vi "test-swerve-drve-odometry-02.vi"() -> (3 "Test Passed":bool)   [LabVIEW 2019]
uses:
  <vilib>/Rock Robotics/WPI/ThirdParty/JAS_Junk/TrajLib/SWERVE_DRIVE_ODOMETRY.ctl
  <vilib>/Rock Robotics/WPI/ThirdParty/JAS_Junk/TrajLib/POSE2D.ctl
  <vilib>/Rock Robotics/WPI/ThirdParty/JAS_Junk/TrajLib/TRANSLATION2D.ctl
  <vilib>/Rock Robotics/WPI/ThirdParty/JAS_Junk/TrajLib/ROTATION2D.ctl
  <vilib>/Rock Robotics/WPI/ThirdParty/JAS_Junk/TrajLib/SWERVE_DRIVE_KINEMATICS.ctl
  <vilib>/Analysis/Matrix/Datatypes/RealMatrix.ctl
  <vilib>/Rock Robotics/WPI/ThirdParty/JAS_Junk/TrajLib/Conv_Deg_Radians.vi
  <vilib>/Rock Robotics/WPI/ThirdParty/JAS_Junk/TrajLib/Rotation_CreateAngle.vi
  <vilib>/Rock Robotics/WPI/ThirdParty/JAS_Junk/TrajLib/Trajectory_Library.lvlib
  <vilib>/Analysis/Matrix/NI_Matrix.lvlib
panel:
  out "SWERVE_DRIVE_KINEMATICS":T1 {"PrevCoR"."Y" format="%14.3f"; "PrevCoR"."X" format="%14.3f"; "Modules"."Y" format="%14.3f"; "Modules"."X" format="%14.3f"}
  out "Odom 1":T4={"POSE"={"TRANSLATION"={"X"=0.0, "Y"=0.0}, "ROTATION"={"VALUE"=0.0, "COS"=1.0, "SIN"=0.0}}, "GyroOffset"={"VALUE"=0.0, "COS"=1.0, "SIN"=0.0}, "PreviousAngle"={"VALUE"=0.0, "COS"=1.0, "SIN"=0.0}, "PrevTime"=0.0} {"PreviousAngle"."SIN" format="%13.4f"; "PreviousAngle"."COS" format="%13.4f"; "PreviousAngle"."VALUE" format="%13.4f"; "GyroOffset"."SIN" format="%13.4f"; "GyroOffset"."COS" format="%13.4f"; "GyroOffset"."VALUE" format="%13.4f"; "POSE"."ROTATION"."SIN" format="%13.4f"; "POSE"."ROTATION"."COS" format="%13.4f"; "POSE"."ROTATION"."VALUE" format="%13.4f"; "POSE"."TRANSLATION"."Y" format="%14.3f"; "POSE"."TRANSLATION"."X" format="%14.3f"}
  out "Odom 0":T4={"POSE"={"TRANSLATION"={"X"=0.0, "Y"=0.0}, "ROTATION"={"VALUE"=0.0, "COS"=1.0, "SIN"=0.0}}, "GyroOffset"={"VALUE"=0.0, "COS"=1.0, "SIN"=0.0}, "PreviousAngle"={"VALUE"=0.0, "COS"=1.0, "SIN"=0.0}, "PrevTime"=0.0} {"PreviousAngle"."SIN" format="%13.4f"; "PreviousAngle"."COS" format="%13.4f"; "PreviousAngle"."VALUE" format="%13.4f"; "GyroOffset"."SIN" format="%13.4f"; "GyroOffset"."COS" format="%13.4f"; "GyroOffset"."VALUE" format="%13.4f"; "POSE"."ROTATION"."SIN" format="%13.4f"; "POSE"."ROTATION"."COS" format="%13.4f"; "POSE"."ROTATION"."VALUE" format="%13.4f"; "POSE"."TRANSLATION"."Y" format="%14.3f"; "POSE"."TRANSLATION"."X" format="%14.3f"}
  out "robot POSE 0":T5={"TRANSLATION"={"X"=0.0, "Y"=0.0}, "ROTATION"={"VALUE"=0.0, "COS"=1.0, "SIN"=0.0}} {"ROTATION"."SIN" format="%13.4f"; "ROTATION"."COS" format="%13.4f"; "ROTATION"."VALUE" format="%13.4f"; "TRANSLATION"."Y" format="%14.3f"; "TRANSLATION"."X" format="%14.3f"}
  out "robot POSE 1":T5={"TRANSLATION"={"X"=0.0, "Y"=0.0}, "ROTATION"={"VALUE"=0.0, "COS"=1.0, "SIN"=0.0}} {"ROTATION"."SIN" format="%13.4f"; "ROTATION"."COS" format="%13.4f"; "ROTATION"."VALUE" format="%13.4f"; "TRANSLATION"."Y" format="%14.3f"; "TRANSLATION"."X" format="%14.3f"}
  out "robot POSE 2":T5={"TRANSLATION"={"X"=0.0, "Y"=0.0}, "ROTATION"={"VALUE"=0.0, "COS"=1.0, "SIN"=0.0}} {"ROTATION"."SIN" format="%13.4f"; "ROTATION"."COS" format="%13.4f"; "ROTATION"."VALUE" format="%13.4f"; "TRANSLATION"."Y" format="%14.3f"; "TRANSLATION"."X" format="%14.3f"}
  out "Odom 2":T4={"POSE"={"TRANSLATION"={"X"=0.0, "Y"=0.0}, "ROTATION"={"VALUE"=0.0, "COS"=1.0, "SIN"=0.0}}, "GyroOffset"={"VALUE"=0.0, "COS"=1.0, "SIN"=0.0}, "PreviousAngle"={"VALUE"=0.0, "COS"=1.0, "SIN"=0.0}, "PrevTime"=0.0} {"PreviousAngle"."SIN" format="%13.4f"; "PreviousAngle"."COS" format="%13.4f"; "PreviousAngle"."VALUE" format="%13.4f"; "GyroOffset"."SIN" format="%13.4f"; "GyroOffset"."COS" format="%13.4f"; "GyroOffset"."VALUE" format="%13.4f"; "POSE"."ROTATION"."SIN" format="%13.4f"; "POSE"."ROTATION"."COS" format="%13.4f"; "POSE"."ROTATION"."VALUE" format="%13.4f"; "POSE"."TRANSLATION"."Y" format="%14.3f"; "POSE"."TRANSLATION"."X" format="%14.3f"}
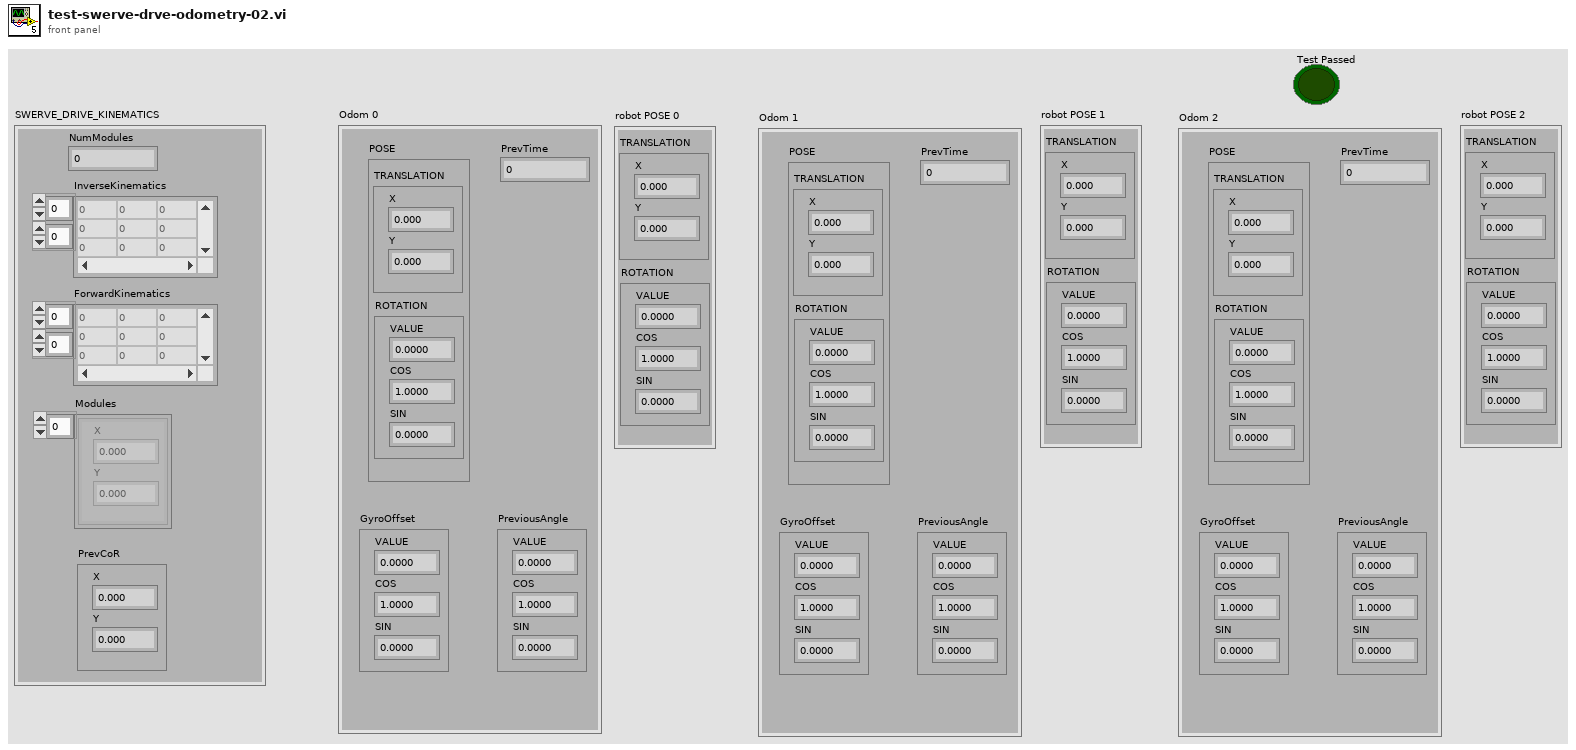
[diagram p1: front panel]
types:
  T1 = typedef "Trajectory_Library.lvlib/SWERVE_DRIVE_KINEMATICS.ctl" = cluster{"NumModules":i32, "InverseKinematics":T2, "ForwardKinematics":T2, "Modules":T3[], "PrevCoR":T3}
  T2 = typedef "NI_Matrix.lvlib/RealMatrix.ctl" = dbl[][]
  T3 = typedef "Trajectory_Library.lvlib/TRANSLATION2D.ctl" = cluster{"X":dbl, "Y":dbl}
  T4 = typedef "Trajectory_Library.lvlib/SWERVE_DRIVE_ODOMETRY.ctl" = cluster{"POSE":T5, "GyroOffset":T6, "PreviousAngle":T6, "PrevTime":dbl}
  T5 = typedef "Trajectory_Library.lvlib/POSE2D.ctl" = cluster{"TRANSLATION":T3, "ROTATION":T6}
  T6 = typedef "Trajectory_Library.lvlib/ROTATION2D.ctl" = cluster{"VALUE":dbl, "COS":dbl, "SIN":dbl}
  T7 = typedef "Trajectory_Library.lvlib/SWERVE_DRIVE_MODULE_STATE.ctl" = cluster{"Speed":dbl, "Angle":T6}
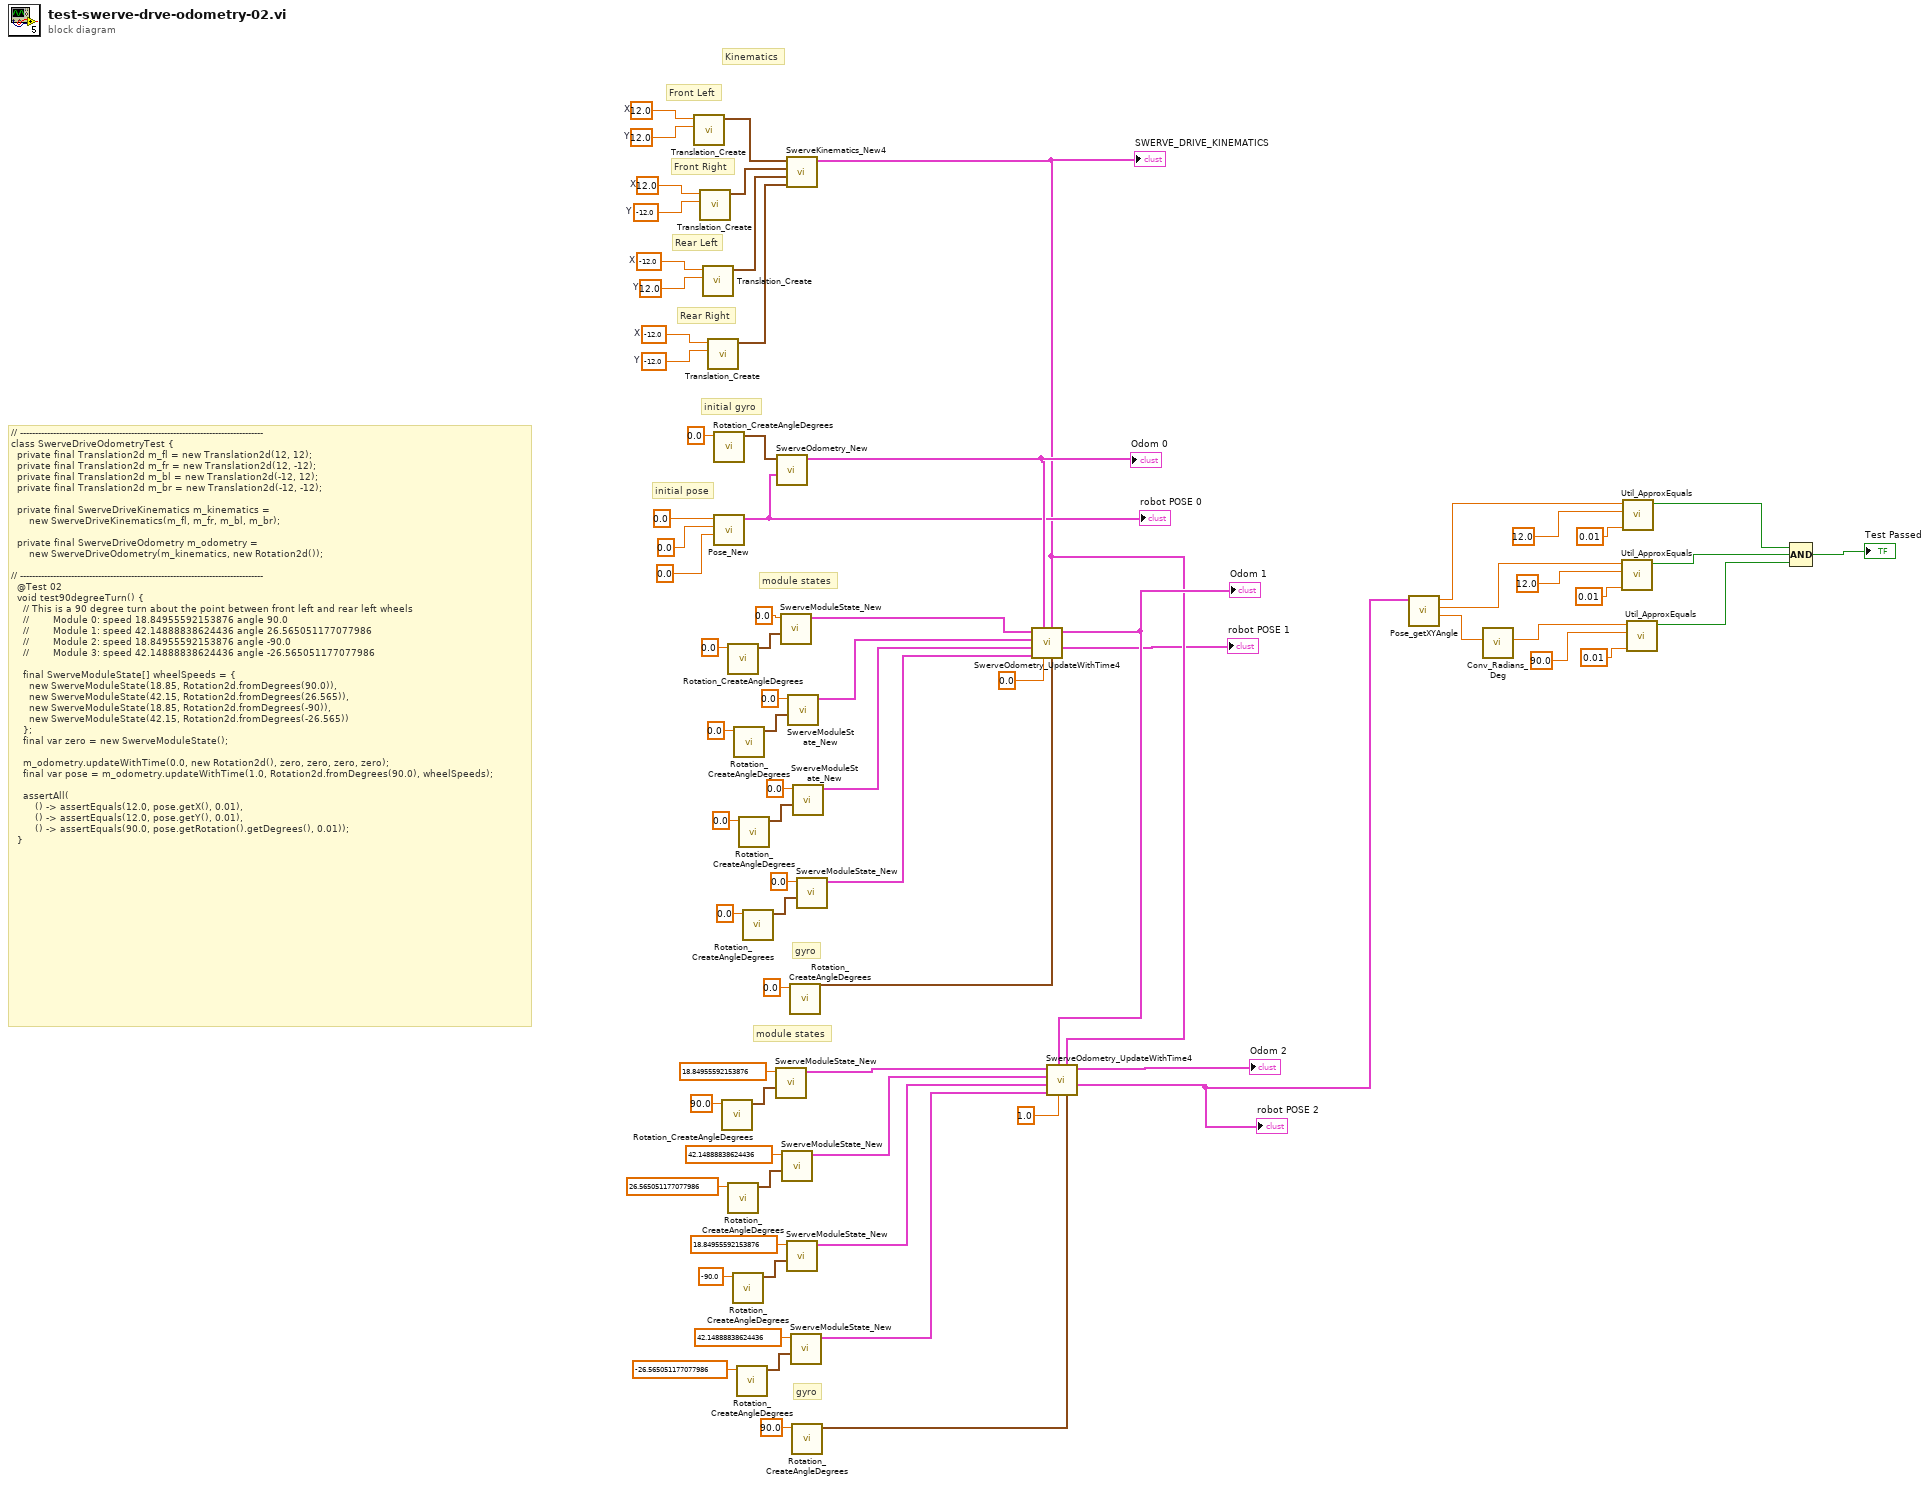
[diagram p0: block diagram]
diagram:
  w72 = -12.0  # X
  w71 = -12.0  # Y
  w70 = -12.0  # X
  w69 = 12.0  # Y
  w68 = 12.0  # X
  w67 = -12.0  # Y
  w66 = 12.0  # X
  w65 = 12.0  # Y
  # "initial pose"
  # "gyro"
  # "module states"
  # "gyro"
  # "module states"
  # "Kinematics"
  # "initial gyro"
  # "Rear Right"
  # "Rear Left"
  # "Front Right"
  # "Front Left"
  # "// ---------------------------------------------------------------------------------\nclass SwerveDriveOdometryTest {\n  private final Translation2d m_fl = new Translation2d(12, 12);\n  private final Translation2d m_fr = new Translation2d(12, -12);\n  private final Translation2d m_bl = new Translation2d(-12, 12);\n  private final Translation2d m_br = new Translation2d(-12, -12);\n\n  private final SwerveDriveKinematics m_kinematics =\n      new SwerveDriveKinematics(m_fl, m_fr, m_bl, m_br);\n\n  private final SwerveDriveOdometry m_odometry =\n      new SwerveDriveOdometry(m_kinematics, new Rotation2d());\n\n// ---------------------------------------------------------------------------------\n  @Test 02\n  void test90degreeTurn() {\n    // This is a 90 degree turn about the point between front left and rear left wheels\n    //        Module 0: speed 18.84955592153876 angle 90.0\n    //        Module 1: speed 42.14888838624436 angle 26.565051177077986\n    //        Module 2: speed 18.84955592153876 angle -90.0\n    //        Module 3: speed 42.14888838624436 angle -26.565051177077986\n\n    final SwerveModuleState[] wheelSpeeds = {\n      new SwerveModuleState(18.85, Rotation2d.fromDegrees(90.0)),\n      new SwerveModuleState(42.15, Rotation2d.fromDegrees(26.565)),\n      new SwerveModuleState(18.85, Rotation2d.fromDegrees(-90)),\n      new SwerveModuleState(42.15, Rotation2d.fromDegrees(-26.565))\n    };\n    final var zero = new SwerveModuleState();\n\n    m_odometry.updateWithTime(0.0, new Rotation2d(), zero, zero, zero, zero);\n    final var pose = m_odometry.updateWithTime(1.0, Rotation2d.fromDegrees(90.0), wheelSpeeds);\n\n    assertAll(\n        () -> assertEquals(12.0, pose.getX(), 0.01),\n        () -> assertEquals(12.0, pose.getY(), 0.01),\n        () -> assertEquals(90.0, pose.getRotation().getDegrees(), 0.01));\n  }"
  n1 = call <vilib>:"Translation_Create.vi"("Y"=w65, "X"=w66) -> ("TRANSLATION"=w73:T3)  [unwired: 9 in]
  n2 = call <vilib>:"Translation_Create.vi"("Y"=w67, "X"=w68) -> ("TRANSLATION"=w74:T3)  [unwired: 9 in]
  n3 = call <vilib>:"Translation_Create.vi"("Y"=w69, "X"=w70) -> ("TRANSLATION"=w75:T3)  [unwired: 9 in]
  n4 = call <vilib>:"Translation_Create.vi"("Y"=w71, "X"=w72) -> ("TRANSLATION"=w76:T3)  [unwired: 9 in]
  n5 = call <vilib>:"Rotation_CreateAngleDegrees.vi"("Angle_Degrees"=0.0) -> ("ROTATION"=w61:T6)  [unwired: 10 in]
  n6 = call <vilib>:"Pose_New.vi"("Heading"=0.0, "Y"=0.0, "X"=0.0) -> ("out POSe"=w28:T5)  [unwired: 8 in]
  "robot POSE 0" <- w28
  n7 = call <vilib>:"Rotation_CreateAngleDegrees.vi"("Angle_Degrees"=90.0) -> ("ROTATION"=w58:T6)  [unwired: 10 in]
  n8 = call <vilib>:"Rotation_CreateAngleDegrees.vi"("Angle_Degrees"=0.0) -> ("ROTATION"=w46:T6)  [unwired: 10 in]
  n9 = call <vilib>:"Rotation_CreateAngleDegrees.vi"("Angle_Degrees"=26.565051177077986) -> ("ROTATION"=w55:T6)  [unwired: 10 in]
  n10 = call <vilib>:"Rotation_CreateAngleDegrees.vi"("Angle_Degrees"=-90.0) -> ("ROTATION"=w52:T6)  [unwired: 10 in]
  n11 = call <vilib>:"Rotation_CreateAngleDegrees.vi"("Angle_Degrees"=0.0) -> ("ROTATION"=w43:T6)  [unwired: 10 in]
  n12 = call <vilib>:"Rotation_CreateAngleDegrees.vi"("Angle_Degrees"=-26.565051177077986) -> ("ROTATION"=w49:T6)  [unwired: 10 in]
  n13 = call <vilib>:"Rotation_CreateAngleDegrees.vi"("Angle_Degrees"=0.0) -> ("ROTATION"=w40:T6)  [unwired: 10 in]
  n14 = call <vilib>:"Rotation_CreateAngleDegrees.vi"("Angle_Degrees"=0.0) -> ("ROTATION"=w37:T6)  [unwired: 10 in]
  n15 = call <vilib>:"SwerveModuleState_New.vi"("ROTATION"=w58, "Speed"=18.84955592153876) -> ("SWERVE_DRIVE_MODULE_STATE"=w4:T7)  [unwired: 9 in]
  n16 = call <vilib>:"SwerveOdometry_New.vi"("InitialPose"=w28, "gyroAngle"=w61) -> ("SWERVE_DRIVE_ODOMETRY"=w29:T4)  [unwired: 9 in]
  "Odom 0" <- w29
  n17 = call <vilib>:"SwerveModuleState_New.vi"("ROTATION"=w46, "Speed"=0.0) -> ("SWERVE_DRIVE_MODULE_STATE"=w8:T7)  [unwired: 9 in]
  n18 = call <vilib>:"SwerveModuleState_New.vi"("ROTATION"=w55, "Speed"=42.14888838624436) -> ("SWERVE_DRIVE_MODULE_STATE"=w3:T7)  [unwired: 9 in]
  n19 = call <vilib>:"SwerveKinematics_New4.vi"("wheel 3"=w76, "wheel 2"=w75, "wheel 1"=w74, "wheel 0"=w73) -> ("SWERVE_DRIVE_KINEMATICS"=w25:T1)  [unwired: 7 in]
  "SWERVE_DRIVE_KINEMATICS" <- w25
  n20 = call <vilib>:"SwerveModuleState_New.vi"("ROTATION"=w52, "Speed"=18.84955592153876) -> ("SWERVE_DRIVE_MODULE_STATE"=w2:T7)  [unwired: 9 in]
  n21 = call <vilib>:"SwerveModuleState_New.vi"("ROTATION"=w43, "Speed"=0.0) -> ("SWERVE_DRIVE_MODULE_STATE"=w7:T7)  [unwired: 9 in]
  n22 = call <vilib>:"Rotation_CreateAngleDegrees.vi"("Angle_Degrees"=0.0) -> ("ROTATION"=w34:T6)  [unwired: 10 in]
  n23 = call <vilib>:"SwerveModuleState_New.vi"("ROTATION"=w49, "Speed"=42.14888838624436) -> ("SWERVE_DRIVE_MODULE_STATE"=w1:T7)  [unwired: 9 in]
  n24 = call <vilib>:"Rotation_CreateAngleDegrees.vi"("Angle_Degrees"=90.0) -> ("ROTATION"=w30:T6)  [unwired: 10 in]
  n25 = call <vilib>:"SwerveModuleState_New.vi"("ROTATION"=w40, "Speed"=0.0) -> ("SWERVE_DRIVE_MODULE_STATE"=w6:T7)  [unwired: 9 in]
  n26 = call <vilib>:"SwerveModuleState_New.vi"("ROTATION"=w37, "Speed"=0.0) -> ("SWERVE_DRIVE_MODULE_STATE"=w5:T7)  [unwired: 9 in]
  n27 = call <vilib>:"SwerveOdometry_UpdateWithTime4.vi"("gyroAngle"=w34, "SWERVE_DRIVE_KINEMATICS"=w25, "Time"=0.0, "in SWERVE_DRIVE_ODOMETRY"=w29, "Wheel State 3"=w5, "Wheel State 2"=w6, "Wheel State 1"=w7, "Wheel State 0"=w8) -> ("robot POSE"=→"robot POSE 1":T5, "out SWERVE_DRIVE_ODOMETRY"=w27:T4)  [unwired: 2 in]
  "Odom 1" <- w27
  n28 = call <vilib>:"SwerveOdometry_UpdateWithTime4.vi"("gyroAngle"=w30, "SWERVE_DRIVE_KINEMATICS"=w25, "Time"=1.0, "in SWERVE_DRIVE_ODOMETRY"=w27, "Wheel State 3"=w1, "Wheel State 2"=w2, "Wheel State 1"=w3, "Wheel State 0"=w4) -> ("robot POSE"=w9:T5, "out SWERVE_DRIVE_ODOMETRY"=→"Odom 2":T4)  [unwired: 2 in]
  "robot POSE 2" <- w9
  n29 = call <vilib>:"Pose_getXYAngle.vi"("in POSE"=w9) -> ("Angle"=w21:dbl, "Y"=w18:dbl, "X"=w19:dbl)  [unwired: 8 in]
  n30 = call <vilib>:"Conv_Radians_Deg.vi"("Radians"=w21) -> ("Degrees"=w17:dbl)  [unwired: 10 in]
  n31 = call <vilib>:"Util_ApproxEquals.vi"("Tolerance"=0.01, "Value 2"=12.0, "Value 1"=w18) -> ("ApproxEquals"=w12:bool)  [unwired: 8 in]
  n32 = call <vilib>:"Util_ApproxEquals.vi"("Tolerance"=0.01, "Value 2"=12.0, "Value 1"=w19) -> ("ApproxEquals"=w13:bool)  [unwired: 8 in]
  n33 = call <vilib>:"Util_ApproxEquals.vi"("Tolerance"=0.01, "Value 2"=90.0, "Value 1"=w17) -> ("ApproxEquals"=w11:bool)  [unwired: 8 in]
  n34 = Compound Arithmetic op=AND(w13, w12, w11) -> (→"Test Passed":bool)
